vi "Saline_monitoring_system.vi"() -> ()   [LabVIEW 2022 SP3]
uses:
  <vilib>/DAQmx/read.llb/DAQmx Read (Digital Bool 1Line 1Point).vi
  <vilib>/DAQmx/read.llb/DAQmx Read (Analog DBL 1Chan 1Samp).vi
  <vilib>/DAQmx/write.llb/DAQmx Write (Digital Bool 1Line 1Point).vi
  <vilib>/Instr/_visa.llb/VISA Configure Serial Port (Instr).vi
  <vilib>/DAQmx/create/channels.llb/DAQmx Create Channel (AI-Voltage-Basic).vi
  <vilib>/DAQmx/create/channels.llb/DAQmx Create Channel (DO-Digital Output).vi
  <vilib>/DAQmx/create/channels.llb/DAQmx Create Channel (DI-Digital Input).vi
  <vilib>/DAQmx/miscellaneous.llb/DAQmx Fill In Error Info.vi
panel:
  out "Buzzer":bool
  out "Boolean Hall Effect":bool
  in  "DAQmx Physical Channel motor":tag
  in  "Hall effect  Input Channel":tag
  in  "Buzzar alarm Output Channel":tag
  out "Boolean Air gap":bool
  out "Waveform Air gap":dbl(graph)
  out "Output Air gap":dbl
  in  "Air Gap detect Channel":tag
  out "Flow rate Meter":dbl(knob) scale=0.0..30.0
  out "Flow rate":dbl
  out "weight":dbl
  out "Liquid Level":dbl(slide) scale=0.0..1000.0
  out "sensor reading":string
  in  "stop":bool
  in  "VISA resource name":refnum<visa-resource-name>
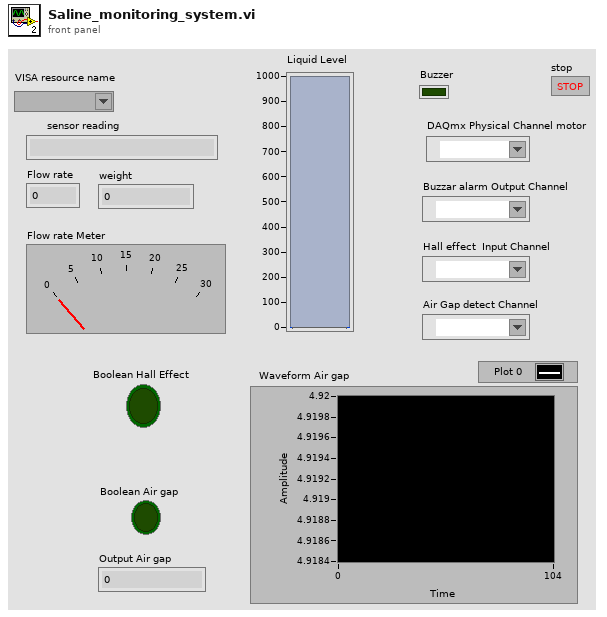
[diagram p1: front panel]
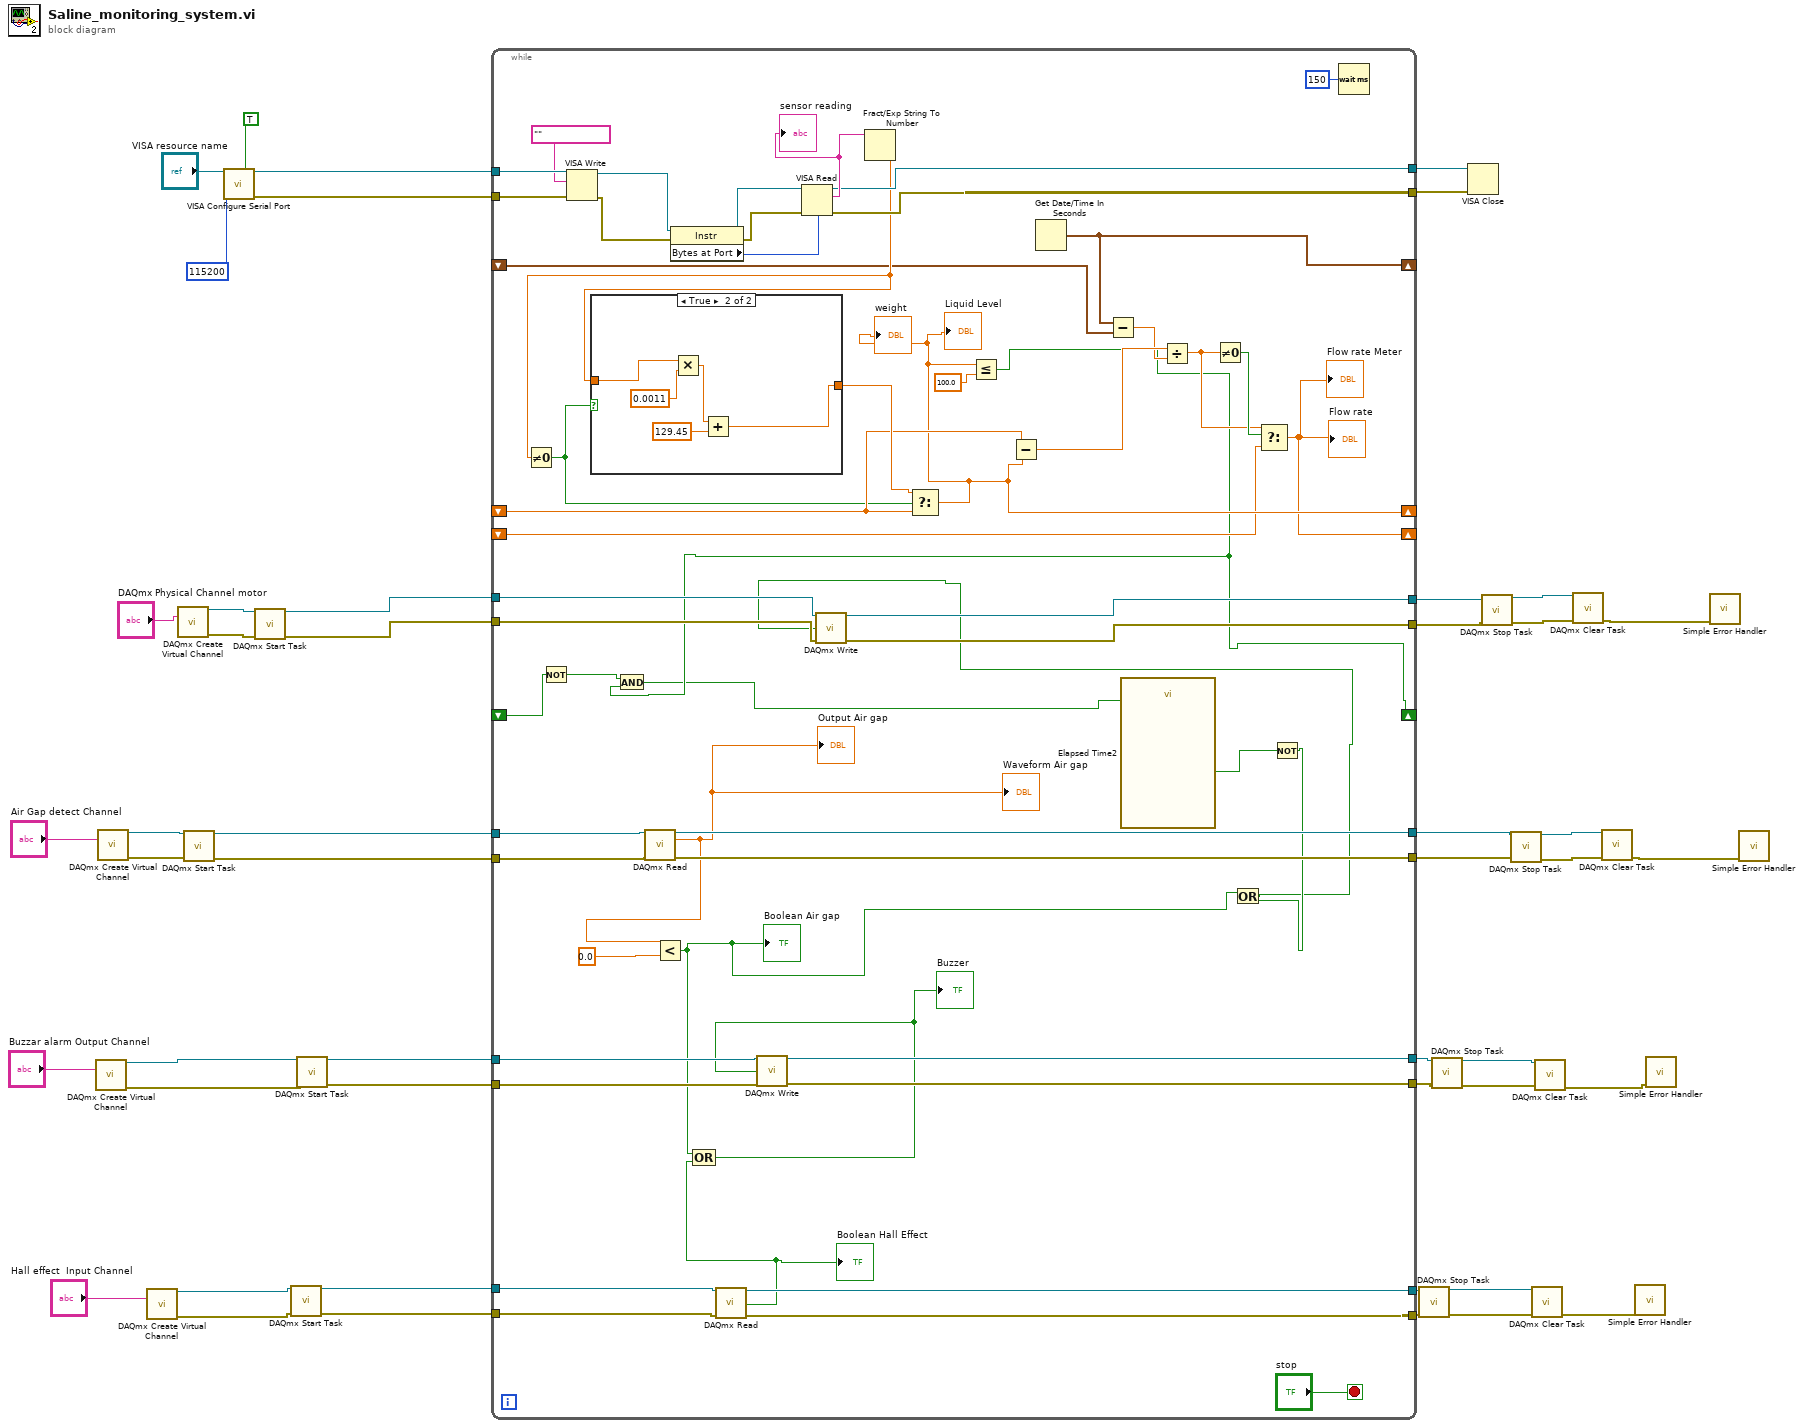
[diagram p0: block diagram]
diagram:
  n1 = call-poly <vilib>:"DAQmx Create Virtual Channel.vi"("lines"="Buzzar alarm Output Channel") -> ("task out"=w29:refnum<k21>, "error out"=w28:errorcluster)  [unwired: 13 in]
  n2 = call-poly <vilib>:"DAQmx Create Virtual Channel.vi"("physical channels"="Air Gap detect Channel") -> ("task out"=w39:refnum<k21>, "error out"=w40:errorcluster)  [unwired: 13 in]
  n3 = call-poly <vilib>:"DAQmx Create Virtual Channel.vi"("lines"="Hall effect  Input Channel") -> ("task out"=w21:refnum<k21>, "error out"=w20:errorcluster)  [unwired: 13 in]
  n4 = call-poly <vilib>:"DAQmx Create Virtual Channel.vi"("lines"="DAQmx Physical Channel motor") -> ("task out"=w10:refnum<k21>, "error out"=w9:errorcluster)  [unwired: 13 in]
  n5 = call <vilib>:"DAQmx Start Task.vi"("task/channels in"=w39, "error in"=w40) -> ("task out"=w34:refnum<k21>, "error out"=w33:errorcluster)  [unwired: 12 in]
  n6 = call-poly "VISA Configure Serial Port"("VISA resource name"="VISA resource name", "Enable Termination\nChar (T)"=TRUE ("Enable Termination\nChar (T)"), "baud rate (9600)"=u32 115200) -> ("VISA resource name out"=w46:refnum<visa-resource-name>, "error out"=w45:errorcluster)  [unwired: 11 in]
  n7 = call <vilib>:"DAQmx Start Task.vi"("task/channels in"=w10, "error in"=w9) -> ("task out"=w2:refnum<k21>, "error out"=w1:errorcluster)  [unwired: 12 in]
  n8 = call <vilib>:"DAQmx Start Task.vi"("task/channels in"=w21, "error in"=w20) -> ("task out"=w16:refnum<k21>, "error out"=w15:errorcluster)  [unwired: 12 in]
  n9 = call <vilib>:"DAQmx Start Task.vi"("task/channels in"=w29, "error in"=w28) -> ("task out"=w18:refnum<k21>, "error out"=w17:errorcluster)  [unwired: 12 in]
  n10 = while {
    tunnel: w46 -> [w102]
    tunnel: w45 -> [w101]
    tunnel: [w90] -> w44
    tunnel: [w92] -> w43
    shift-right: [w82] -> _
    shift-left: _ -> [w83]
    shift-right: [w87] -> _
    shift-left: _ -> [w86]
    shift-right: [w64] -> _
    shift-left: _ -> [w80]
    tunnel: w34 -> [w77]
    tunnel: w33 -> [w76]
    tunnel: [w75] -> w32
    tunnel: [w74] -> w31
    tunnel: w18 -> [w73]
    tunnel: w17 -> [w72]
    tunnel: w16 -> [w71]
    tunnel: w15 -> [w70]
    tunnel: [w69] -> w14
    tunnel: [w68] -> w13
    tunnel: [w67] -> w12
    tunnel: [w66] -> w11
    tunnel: [w61] -> w4
    tunnel: [w60] -> w3
    tunnel: w2 -> [w59]
    tunnel: w1 -> [w58]
    shift-right: [w55] -> _
    shift-left: _ -> [w57]
    stop <- "stop" stop-if-true
    n11 = Not(x=w57) -> (.not. x?=w56:bool)
    n12 = VISA Write(VISA resource name=w102, write buffer="", error in (no error)=w101) -> (VISA resource name out=w100:refnum<visa-resource-name>, error out=w99:errorcluster)  [unwired: 1 out]
    n13 = call-poly <vilib>:"DAQmx Read.vi"("task/channels in"=w77, "error in"=w76) -> ("task out"=w75:refnum<k21>, "data"=w63:dbl, "error out"=w74:errorcluster)  [unwired: 11 in]
    "Output Air gap" <- w63
    "Waveform Air gap" <- w63
    n14 = Less?(x=w63, y=0.0) -> (x < y?=w50:bool)
    "Boolean Air gap" <- w50
    n15 = property class="Instr"(reference=w100, error in=w99) -> (reference out=w93:refnum<visa-resource-name>, error out=w94:errorcluster, "Bytes at Port"=w95:u32)
    n16 = call-poly <vilib>:"DAQmx Read.vi"("task/channels in"=w71, "error in"=w70) -> ("task out"=w69:refnum<k21>, "data"=w52:bool, "error out"=w68:errorcluster)  [unwired: 11 in]
    "Boolean Hall Effect" <- w52
    n17 = Compound Arithmetic op=OR(w50, w52) -> (w51:bool)
    "Buzzer" <- w51
    n18 = call-poly <vilib>:"DAQmx Write.vi"("task/channels in"=w73, "data"=w51, "error in"=w72) -> ("task out"=w67:refnum<k21>, "error out"=w66:errorcluster)  [unwired: 10 in, 1 out]
    n19 = VISA Read(VISA resource name=w93, byte count=w95, error in (no error)=w94) -> (VISA resource name out=w90:refnum<visa-resource-name>, read buffer=w91:string, error out=w92:errorcluster)  [unwired: 1 out]
    "sensor reading" <- w91
    n20 = Fract/Exp String To Number(string=w91) -> (number=w89:dbl)  [unwired: 3 in, 1 out]
    n21 = Not Equal To 0?(x=w89) -> (x != 0?=w65:bool)
    n22 = case shown="True" w65 {
      tunnel: w89 -> [w103 w107]
      tunnel: [w103 w104] -> w88
      frame False {
      }
      frame True {
        n23 = Multiply(x=w107, y=0.0011) -> (x*y=w105:dbl)
        n24 = Add(x=w105, y=129.45) -> (x+y=w104:dbl)
      }
    }
    n25 = Select(t=w88, s=w65, f=w83) -> (s? t:f=w82:dbl)
    "weight" <- w82
    "Liquid Level" <- w82
    n26 = Less Or Equal?(x=w82, y=100.0) -> (x <= y?=w55:bool)
    n27 = And(x=w56, y=w55) -> (x .and. y?=w54:bool)
    n28 = Subtract(x=w83, y=w82) -> (x-y=w85:dbl)
    n29 = Get Date/Time In Seconds() -> (seconds since 1Jan1904=w87:timestamp)
    n30 = Subtract(x=w87, y=w86) -> (x-y=w84:dbl)
    n31 = call "Elapsed Time2"("Reset"=w54) -> ("Time has Elapsed"=w53:bool)  [unwired: 11 in, 7 out]
    n32 = Divide(x=w85, y=w84) -> (x/y=w79:dbl)
    n33 = Not Equal To 0?(x=w79) -> (x != 0?=w81:bool)
    n34 = Select(t=w79, s=w81, f=w80) -> (s? t:f=w64:dbl)
    "Flow rate" <- w64
    "Flow rate Meter" <- w64
    n35 = Not(x=w53) -> (.not. x?=w49:bool)
    n36 = Or(x=w50, y=w49) -> (x .or. y?=w48:bool)
    n37 = call-poly <vilib>:"DAQmx Write.vi"("task/channels in"=w59, "data"=w48, "error in"=w58) -> ("task out"=w61:refnum<k21>, "error out"=w60:errorcluster)  [unwired: 10 in, 1 out]
    n38 = Wait (ms)(milliseconds to wait=u32 150) -> ()  [unwired: 1 out]
  }
  n39 = call <vilib>:"DAQmx Stop Task.vi"("task/channels in"=w14, "error in"=w13) -> ("task out"=w27:refnum<k21>, "error out"=w26:errorcluster)  [unwired: 12 in]
  n40 = call <vilib>:"DAQmx Stop Task.vi"("task/channels in"=w12, "error in"=w11) -> ("task out"=w25:refnum<k21>, "error out"=w24:errorcluster)  [unwired: 12 in]
  n41 = VISA Close(VISA resource name=w44, error in (no error)=w43) -> ()  [unwired: 1 out]
  n42 = call <vilib>:"DAQmx Stop Task.vi"("task/channels in"=w4, "error in"=w3) -> ("task out"=w7:refnum<k21>, "error out"=w6:errorcluster)  [unwired: 12 in]
  n43 = call <vilib>:"DAQmx Stop Task.vi"("task/channels in"=w32, "error in"=w31) -> ("task out"=w37:refnum<k21>, "error out"=w36:errorcluster)  [unwired: 12 in]
  n44 = call <vilib>:"DAQmx Clear Task.vi"("task in"=w27, "error in"=w26) -> ("error out"=w22:errorcluster)  [unwired: 13 in]
  n45 = call <vilib>:"DAQmx Clear Task.vi"("task in"=w25, "error in"=w24) -> ("error out"=w23:errorcluster)  [unwired: 13 in]
  n46 = call <vilib>:"DAQmx Clear Task.vi"("task in"=w7, "error in"=w6) -> ("error out"=w5:errorcluster)  [unwired: 13 in]
  n47 = call <vilib>:"DAQmx Clear Task.vi"("task in"=w37, "error in"=w36) -> ("error out"=w35:errorcluster)  [unwired: 13 in]
  n48 = call <vilib>:"Simple Error Handler.vi"("error in (no error)"=w22) -> ()  [unwired: 4 in, 5 out]
  n49 = call <vilib>:"Simple Error Handler.vi"("error in (no error)"=w23) -> ()  [unwired: 4 in, 5 out]
  n50 = call <vilib>:"Simple Error Handler.vi"("error in (no error)"=w5) -> ()  [unwired: 4 in, 5 out]
  n51 = call <vilib>:"Simple Error Handler.vi"("error in (no error)"=w35) -> ()  [unwired: 4 in, 5 out]
